vi "BRig_RT__Case_Exp__recordAnalogInput__PortC.vi"(0 "input_dataAnalog":u16[][](array[numeric]), 1 "input_index":i32, 2 "input_iOccurence":u16, 3 "resetOccurrence":bool, 4 "input_dataCurrent":u16[](array[numeric]), 5 "input_prevStorage":bool, 6 "input_iState_start":T1, 7 "input_stateList_NoInterrupt":u16[](array[numeric]), 8 "input_iState_end":T1, 10 "input_AI1":i16, 12 "input_AI0":i16) -> (14 "output_dataAnalog":u16[][](array[numeric]), 15 "output_index":i32, 16 "output_iOccurrence":u16, 19 "output_prevStorage":bool)   [LabVIEW 2014]
uses:
  myRIO_BRig_RT__Case_Exp_stateList.ctl
  <vilib>/Utility/file.llb/Write To Spreadsheet File (DBL).vi
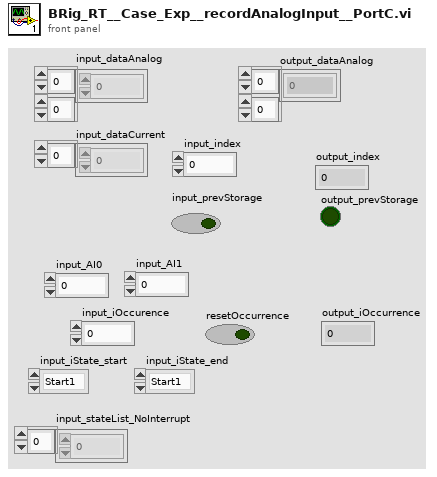
[diagram p1: front panel]
types:
  T1 = typedef "myRIO_BRig_RT__Case_Exp_stateList.ctl" = enum16{"Start1", "Start2", "Start3", "saveSettings1", "saveSettings2", "saveSettings3", "saveSettings4", "saveSettings_LC_ENL_l1", "saveSettings_LC_ENL_l2", "saveSettings_LC_Cue_l1", "saveSettings_LC_Cue_l2", "saveSettings6_LC_l1_Other", "SaveSettings6_LC_l2_Other", "setSettings_Audio", "setSettings_Laser", "initBlock_pre", "initBlock", "initBlock2", "initBlock_post", "initTrial_pre", "initTrial", "initTrial2", "initTrial3", "initTrial4", "initTrial_LC_ENL1", "initTrial_LC_Cue1", "initTrial_LC_Cue1_2", "initTrial_LC_Sel", "initTrial_post", "ENL1_pre", "ENL1", "ENL1_post", "ENL1Penalty_pre", "ENL1Penalty", "ENL2_pre", "ENL2", "ENL2Penalty_pre", "ENL2Penalty", "Cue1_pre", "Cue1", "Cue1_post", "Cue1Penalty_pre", "Cue1Penalty", "Cue2_pre", "Cue2", "Cue2Penalty_pre", "Cue2Penalty", "Selection_pre", "Selection", "Select_post", "SelectReward_pre", "SelectReward", "SelectRewardPost_pre", "SelectRewardPost", "SelectWrong_pre", "SelectWrong", "SelectWrong_post", "SelectTimeout_pre", "SelectTimeout", "SelectTimeout_post", "endTrial_pre", "endTrial1", "endTrial2", "endTrial3", "endTrial_post", "endBlock_pre", "endBlock", "endBlock_post", "endExp", "commConnect", "commUpload_pre", "commUpload_dataBlock", "commUpload_dataCurrent", "commUpload_dataExp", "commUpload_dataLC", "commUpload_dataTrial", "commUpload_post", "saveData_pre", "saveData_dataBlock", "saveData_dataCurrent", "saveData_dataExp", "saveData_dataLC", "saveData_dataTrial", "saveData_post", "empty_endBlock1", "empty_endBlock2", "empty_endTrial1", "empty_endTrial2", "empty_endTrial3", "empty_endTrial4", "empty_endTrial5", "dummyState", "dummyState_endBlock", "FreeReward_pre", "FreeReward", "FreeRewardPost_pre", "FreeRewardPost"}
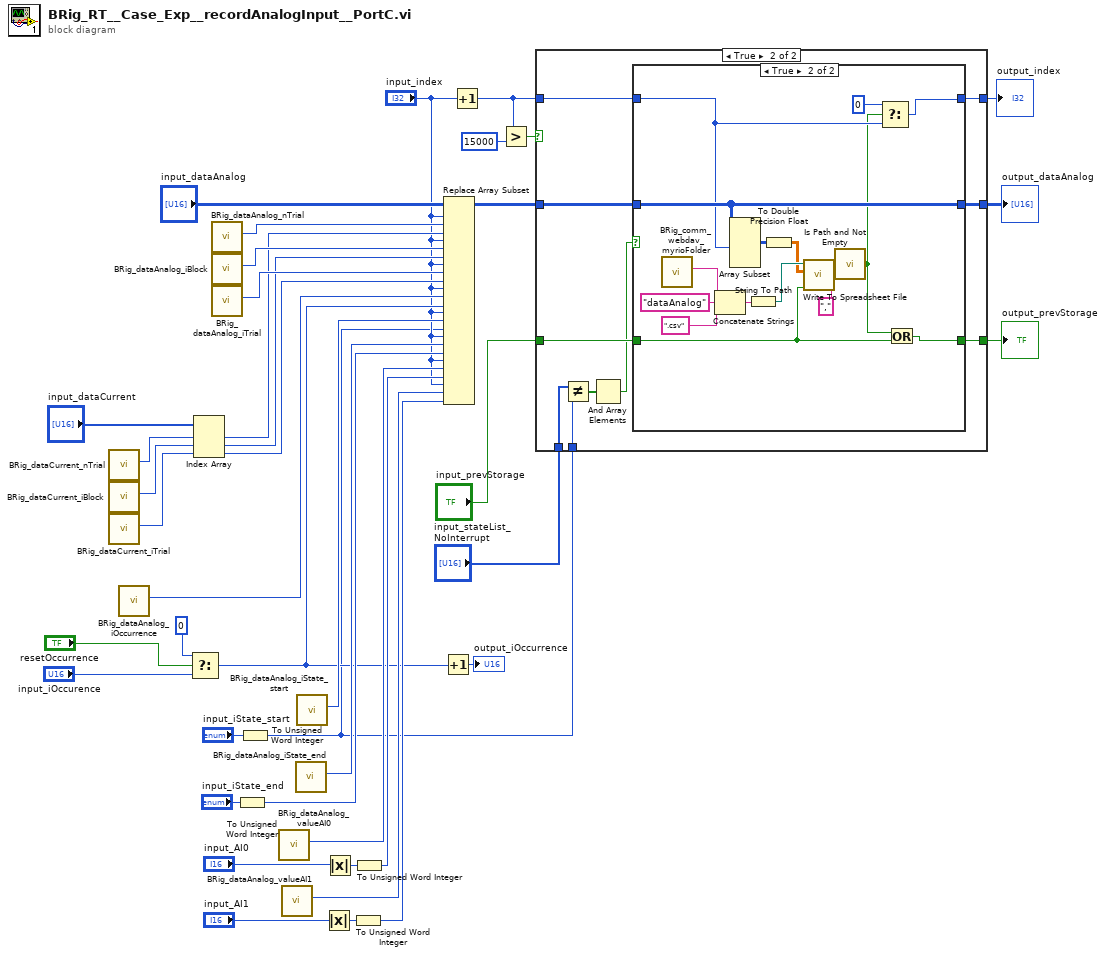
[diagram p0: block diagram]
diagram:
  n1 = call "BRig_dataCurrent_nTrial.vi"() -> ("output_nTrial"=w37:i32)  [unwired: 11 in]
  n2 = call "BRig_dataCurrent_iBlock.vi"() -> ("output_iBlock"=w36:i32)  [unwired: 11 in]
  n3 = call "BRig_dataCurrent_iTrial.vi"() -> ("output_iTrial"=w35:i32)  [unwired: 11 in]
  n4 = call "BRig_dataAnalog_iOccurrence.vi"() -> ("output_iOccurrence"=w28:i32)  [unwired: 11 in]
  n5 = Select(t=u16 0, s="resetOccurrence", f="input_iOccurence") -> (s? t:f=w19:u16)
  n6 = Index Array(array="input_dataCurrent", index #1=w37, index #2=w36, index #3=w35) -> (element #1=w13:u16, element #2=w14:u16, element #3=w12:u16)
  n7 = call "BRig_dataAnalog_nTrial.vi"() -> ("output_nTrial"=w34:i32)  [unwired: 11 in]
  n8 = call "BRig_dataAnalog_iBlock.vi"() -> ("output_iBlock"=w33:i32)  [unwired: 11 in]
  n9 = call "BRig_dataAnalog_iTrial.vi"() -> ("output_iTrial"=w32:i32)  [unwired: 11 in]
  n10 = To Unsigned Word Integer(number="input_iState_end") -> (unsigned 16bit integer=w27:u16)
  n11 = To Unsigned Word Integer(number="input_iState_start") -> (unsigned 16bit integer=w2:u16)
  n12 = call "BRig_dataAnalog_valueAI0.vi"() -> ("output_valueAI0"=w26:i32)  [unwired: 11 in]
  n13 = call "BRig_dataAnalog_valueAI1.vi"() -> ("output_valueAI1"=w25:i32)  [unwired: 11 in]
  n14 = call "BRig_dataAnalog_iState_end.vi"() -> ("output_iState_end"=w29:i32)  [unwired: 11 in]
  n15 = call "BRig_dataAnalog_iState_start.vi"() -> ("output_iState_start"=w30:i32)  [unwired: 11 in]
  n16 = Absolute Value(x="input_AI1") -> (abs(x)=w39:i16)
  n17 = Absolute Value(x="input_AI0") -> (abs(x)=w40:i16)
  n18 = To Unsigned Word Integer(number=w39) -> (unsigned 16bit integer=w23:u16)
  n19 = To Unsigned Word Integer(number=w40) -> (unsigned 16bit integer=w24:u16)
  n20 = Increment(x=w19) -> (x+1=→"output_iOccurrence":u16)
  n21 = Replace Array Subset(array="input_dataAnalog", new element #1=w13, index (row) #1="input_index", index (col) #1=w34, new element #2=w14, index (row) #2="input_index", index (col) #2=w33, new element #3=w12, index (row) #3="input_index", index (col) #3=w32, new element #4=w19, index (row) #4="input_index", index (col) #4=w28, new element #5=w2, index (row) #5="input_index", index (col) #5=w30, new element #6=w27, index (row) #6="input_index", index (col) #6=w29, new element #7=w24, index (row) #7="input_index", index (col) #7=w26, new element #8=w23, index (row) #8="input_index", index (col) #8=w25) -> (w8:u16[][])
  n22 = Increment(x="input_index") -> (x+1=w7:i32)
  n23 = Greater?(x=w7, y=15000) -> (0:w9:bool)
  n24 = case shown="True" w9 {
    tunnel: w8 -> [w44 w53]
    tunnel: [w44 w53] -> w6
    tunnel: w7 -> [w43 w52]
    tunnel: [w43 w51] -> w5
    tunnel: "input_prevStorage" -> [w42 w50]
    tunnel: [w42 w49] -> w3
    tunnel: w2 -> [_ w47]
    tunnel: "input_stateList_NoInterrupt" -> [_ w48]
    frame False {
    }
    frame True {
      n25 = Not Equal?(x=w48, y=w47) -> (x != y?=w46:bool[])
      n26 = And Array Elements(Boolean array=w46) -> (logical AND=w45:bool)
      n27 = case shown="True" w45 {
        tunnel: w53 -> [w55 w57]
        tunnel: w52 -> [w56 w63]
        tunnel: [w56 w61] -> w51
        tunnel: w50 -> [w54 w59]
        tunnel: [w54 w58] -> w49
        tunnel: [w55 w57] -> _
        frame False {
        }
        frame True {
          n28 = call "BRig_comm_webdav_myrioFolder.vi"() -> ("output_myrioFolder"=w72:string)  [unwired: 11 in]
          n29 = Concatenate Strings(w72, "dataAnalog" ("input_filename"), ".csv" ("string")) -> (w70:string)
          n30 = Array Subset(array=w57, length (row)=w63) -> (w68:u16[][])  [unwired: 3 in]
          n31 = String To Path(string=w70) -> (path=w65:path)
          n32 = To Double Precision Float(number=w68) -> (double precision float=w64:dbl[][])
          n33 = call-poly <vilib>:"Write To Spreadsheet File.vi"("delimiter (\\t)"="," ("delimiter (\\t)"), "append to file? (new file:F)"=w59, "2D data"=w64, "file path (dialog if empty)"=w65) -> ("new file path (Not A Path if cancelled)"=w66:path)  [unwired: 4 in]
          n34 = call <vilib>:"Is Path and Not Empty.vi"("path"=w66) -> ("Is Path and Not Empty?"=w60:bool)  [unwired: 4 in]
          n35 = Select(t=0, s=w60, f=w63) -> (s? t:f=w61:i32)
          n36 = Or(x=w60, y=w59) -> (x .or. y?=w58:bool)
        }
      }
    }
  }
  "output_dataAnalog" <- w6
  "output_index" <- w5
  "output_prevStorage" <- w3
